vi "Hide Animated Busy Icon.vi"(2 "Error In":errorcluster) -> (7 "Error Out":errorcluster)   [LabVIEW 2021, in "GUI.lvlib"]
doc: "This VI passes error in through and ignores it."
uses:
  GUI/GUI.lvlib
  Error/Error.lvlib
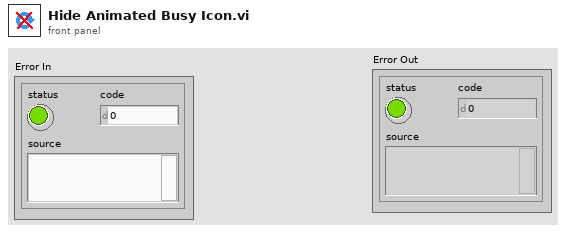
[diagram p1: front panel]
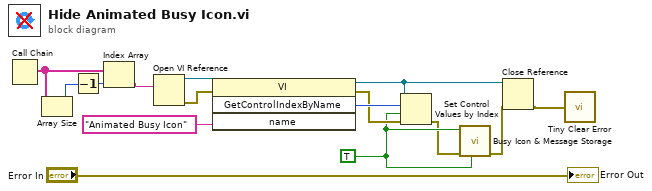
[diagram p0: block diagram]
diagram:
  w3 = TRUE
  n1 = Call Chain() -> (call chain=w15:string[])
  n2 = Array Size(array=w15) -> (size(s)=w14:i32)
  n3 = Decrement(x=w14) -> (x-1=w13:i32)
  n4 = Index Array(array=w15, index=w13) -> (element=w12:string)
  n5 = Open VI Reference(vi path=w12) -> (vi reference=w8:refnum<vi>, error out=w7:errorcluster)  [unwired: 5 in]
  n6 = invoke class="VI" method="GetControlIndexByName"(reference=w8, error in=w7, "name"="Animated Busy Icon" ("element")) -> (reference out=w6:refnum<vi>, error out=w9:errorcluster, "GetControlIndexByName"=w10:i32)  [unwired: 1 in, 1 out]
  n7 = Set Control Values by Index(0:w6, 1:w10, 2:w3, 3:w9) -> (11:w2:errorcluster)
  n8 = call "Busy Icon & Message Storage.vi"("Get(F)/Set Busy Icon"=w3, "Error In"=w2, "Busy Icon Status (F = busy)"=w3) -> ("Error Out"=w1:errorcluster)  [unwired: 6 in, 2 out]
  n9 = Close Reference(reference=w6, error in (no error)=w1) -> (error out=w4:errorcluster)
  n10 = call "Tiny Clear Error.vi"("Error In"=w4) -> ()  [unwired: 8 in, 1 out]
  "Error Out" <- "Error In"
